vi "HeMinSpecForm.vi"() -> ()   [LabVIEW 2012]
panel:
  in  "Cancel Button":bool
  in  "OK Button":bool
  in  "Sm147StoppingDistance":dbl caption="Sm-147 Stopping Distance:"
  in  "Th232StoppingDistance":dbl caption="Th-232 Stopping Distance:"
  in  "U235StoppingDistance":dbl caption="U-235 Stopping Distance:"
  in  "U238StoppingDistance":dbl caption="U-238 Stopping Distance:"
  in  "MineralName":string caption="Mineral Name:"
  # "µm"
  # "µm"
  # "µm"
  # "µm"
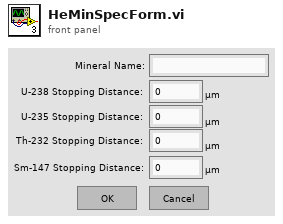
[diagram p1: front panel]
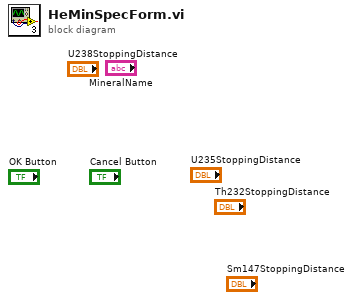
[diagram p0: block diagram]
diagram:
